vi "StopWatch.vi"(2 "Global In (s)":dbl, 3 "Reset Button":bool, 4 "Elapsed In (s)":dbl format="%#_17f") -> (0 "Global Out (s)":dbl, 1 "Elapsed Time (Secs)":dbl)   [LabVIEW 2025]
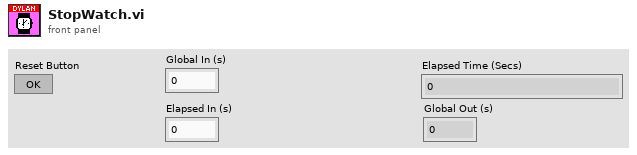
[diagram p1: front panel]
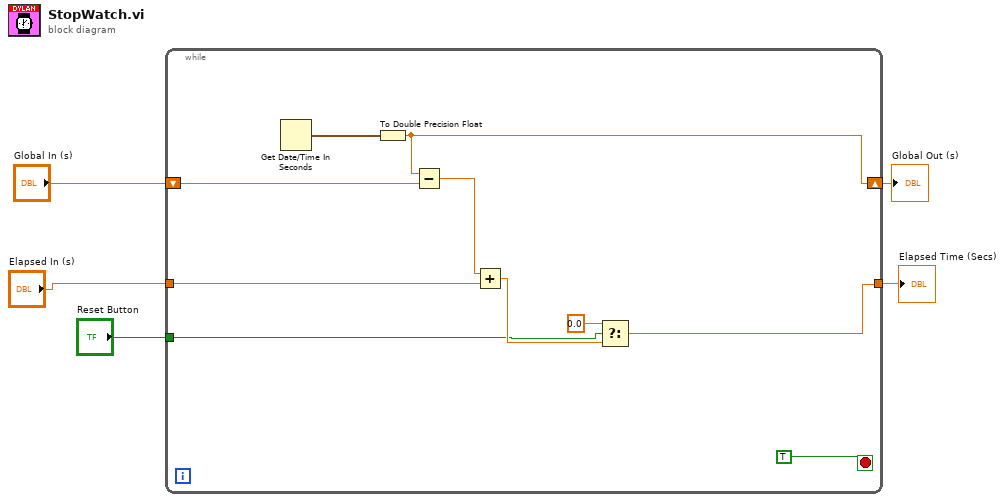
[diagram p0: block diagram]
diagram:
  n1 = while {
    shift-right: [w14] -> w1
    shift-left: "Global In (s)" -> [w6]
    tunnel: "Reset Button" -> [w9]
    tunnel: [w8] -> w4
    tunnel: "Elapsed In (s)" -> [w7]
    stop <- TRUE stop-if-true
    n2 = Get Date/Time In Seconds() -> (seconds since 1Jan1904=w15:timestamp)
    n3 = To Double Precision Float(number=w15) -> (double precision float=w14:dbl)
    n4 = Subtract(x=w14, y=w6) -> (x-y=w13:dbl)
    n5 = Add(x=w13, y=w7) -> (x+y=w10:dbl)
    n6 = Select(t=0.0, s=w9, f=w10) -> (s? t:f=w8:dbl)
  }
  "Elapsed Time (Secs)" <- w4
  "Global Out (s)" <- w1
